vi "ReadDigInterface.vi"(7 "error in":errorcluster, 9 "ON/OFF":bool, 10 "VISA resource name in":refnum<visa-resource-name>) -> (0 "error out":errorcluster, 2 "Extend Device Status":T1, 3 "VISA resource name out":refnum<visa-resource-name>)   [LabVIEW 2014]
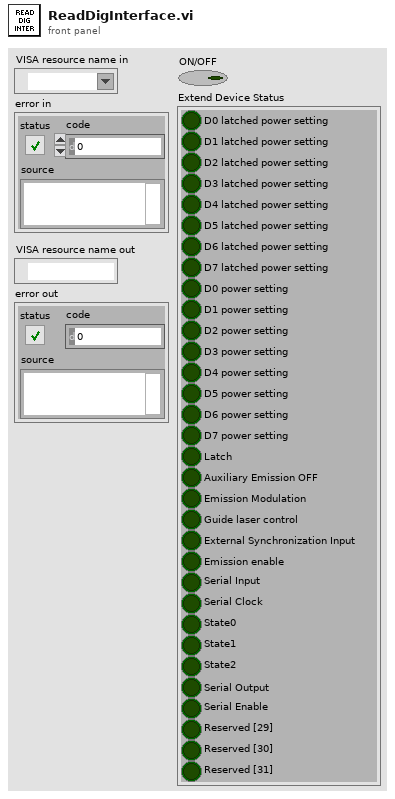
[diagram p1: front panel]
types:
  T1 = cluster{"D0 latched power setting":bool, "D1 latched power setting":bool, "D2 latched power setting":bool, "D3 latched power setting":bool, "D4 latched power setting":bool, "D5 latched power setting":bool, "D6 latched power setting":bool, "D7 latched power setting":bool, "D0 power setting":bool, "D1 power setting":bool, "D2 power setting":bool, "D3 power setting":bool, "D4 power setting":bool, "D5 power setting":bool, "D6 power setting":bool, "D7 power setting":bool, "Latch":bool, "Auxiliary Emission OFF":bool, "Emission Modulation":bool, "Guide laser control":bool, "External Synchronization Input":bool, "Emission enable":bool, "Serial Input":bool, "Serial Clock":bool, "State0":bool, "State1":bool, "State2":bool, "Serial Output":bool, "Serial Enable":bool, "Reserved [29]":bool, "Reserved [30]":bool, "Reserved [31]":bool}
  T2 = cluster{"Boolean array[0]":bool, "Boolean array[1]":bool, "Boolean array[2]":bool, "Boolean array[3]":bool, "Boolean array[4]":bool, "Boolean array[5]":bool, "Boolean array[6]":bool, "Boolean array[7]":bool, "Boolean array[8]":bool, "Boolean array[9]":bool, "Boolean array[10]":bool, "Boolean array[11]":bool, "Boolean array[12]":bool, "Boolean array[13]":bool, "Boolean array[14]":bool, "Boolean array[15]":bool, "Boolean array[16]":bool, "Boolean array[17]":bool, "Boolean array[18]":bool, "Boolean array[19]":bool, "Boolean array[20]":bool, "Boolean array[21]":bool, "Boolean array[22]":bool, "Boolean array[23]":bool, "Boolean array[24]":bool, "Boolean array[25]":bool, "Boolean array[26]":bool, "Boolean array[27]":bool, "Boolean array[28]":bool, "Boolean array[29]":bool, "Boolean array[30]":bool, "Boolean array[31]":bool}
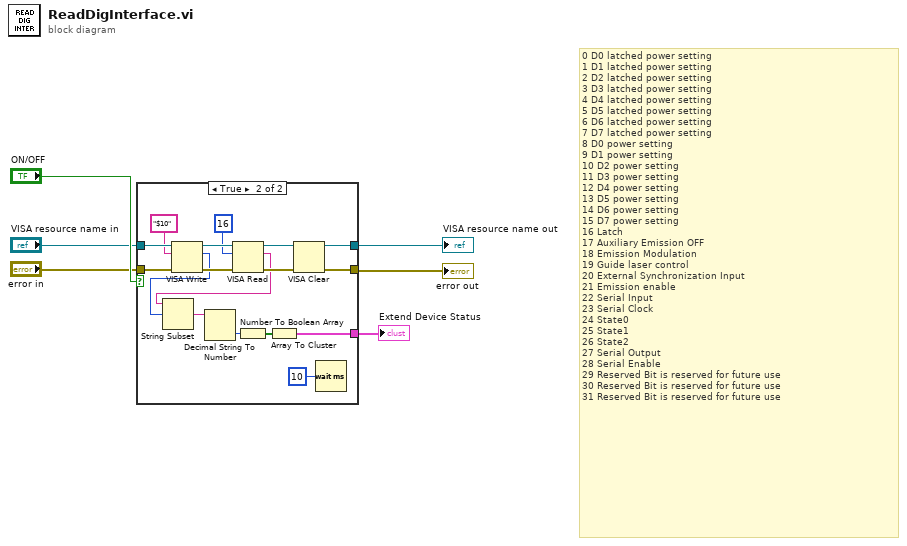
[diagram p0: block diagram]
diagram:
  # "0 D0 latched power setting\n1 D1 latched power setting\n2 D2 latched power setting\n3 D3 latched power setting\n4 D4 latched power setting\n5 D5 latched power setting\n6 D6 latched power setting\n7 D7 latched power setting\n8 D0 power setting\n9 D1 power setting\n10 D2 power setting\n11 D3 power setting\n12 D4 power setting\n13 D5 power setting\n14 D6 power setting\n15 D7 power setting\n16 Latch\n17 Auxiliary Emission OFF\n18 Emission Modulation\n19 Guide laser control\n20 External Synchronization Input\n21 Emission enable\n22 Serial Input\n23 Serial Clock\n24 State0\n25 State1\n26 State2\n27 Serial Output\n28 Serial Enable\n29 Reserved Bit is reserved for future use\n30 Reserved Bit is reserved for future use\n31 Reserved Bit is reserved for future use"
  n1 = case shown="True" "ON/OFF" {
    tunnel: "VISA resource name in" -> [w8 w23]
    tunnel: "error in" -> [w7 w22]
    tunnel: [w8 w19] -> w3
    tunnel: [w7 w18] -> w2
    tunnel: [_ w10] -> w1
    frame False {
    }
    frame True {
      n2 = VISA Write(VISA resource name=w23, write buffer="$10", error in (no error)=w22) -> (VISA resource name out=w24:refnum<visa-resource-name>, return count=w12:u32, error out=w25:errorcluster)
      n3 = VISA Read(VISA resource name=w24, byte count=u32 16, error in (no error)=w25) -> (VISA resource name out=w21:refnum<visa-resource-name>, read buffer=w13:string, error out=w20:errorcluster)  [unwired: 1 out]
      n4 = String Subset(string=w13, offset (0)=w12) -> (substring=w14:string)  [unwired: 1 in]
      n5 = Decimal String To Number(string=w14) -> (number=w15:i32)  [unwired: 2 in, 1 out]
      n6 = Number To Boolean Array(number=w15) -> (Boolean array=w11:bool[])
      n7 = Array To Cluster(array=w11) -> (cluster=w10:T2)
      n8 = VISA Clear(VISA resource name=w21, error in (no error)=w20) -> (VISA resource name out=w19:refnum<visa-resource-name>, error out=w18:errorcluster)
      n9 = Wait (ms)(milliseconds to wait=u32 10) -> ()  [unwired: 1 out]
    }
  }
  "Extend Device Status" <- w1
  "VISA resource name out" <- w3
  "error out" <- w2
